vi "Create TXRX Bytes.vi"(0 "Cluster Array in":T1[](array[typedef]) {"payload" format="%x"; "timestamp" format="%<%.7X\n%x>T"; "type" items=["CAN Data"=0, "CAN Remote"=1, "CAN Bus Error"=2, "CAN 2.0 Data"=8, "CAN FD Data"=16, "CAN FD+BRS Data"=24, "J1939 Data"=192, "Delay"=224, "Log Trigger"=225, "Start Trigger"=226]; "identifier" format="%x"}, 1 "Tx?":bool) -> (7 "Array":string[](array[string]), 8 "Flow Control?":bool, 9 "Block Size":u16 format="%.0x")   [LabVIEW 2018]
uses:
  <vilib>/xnet/xnet.llb/XNET Frame CAN.ctl
  <vilib>/xnet/xnet.llb/XNET Frame Type CAN.ctl
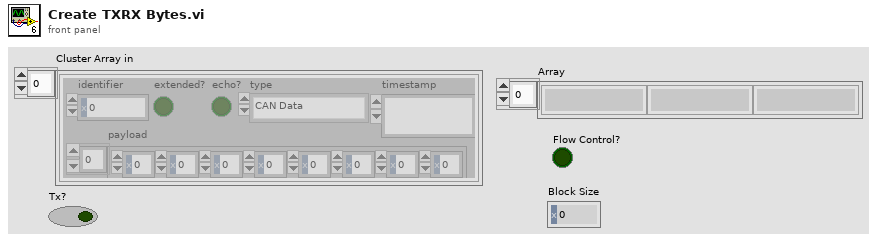
[diagram p1: front panel]
types:
  T1 = typedef "XNET Frame CAN.ctl" = cluster{"timestamp":timestamp, "payload":u8[], "identifier":u32, "type":T2, "extended?":bool, "echo?":bool}
  T2 = typedef "XNET Frame Type CAN.ctl" = u8
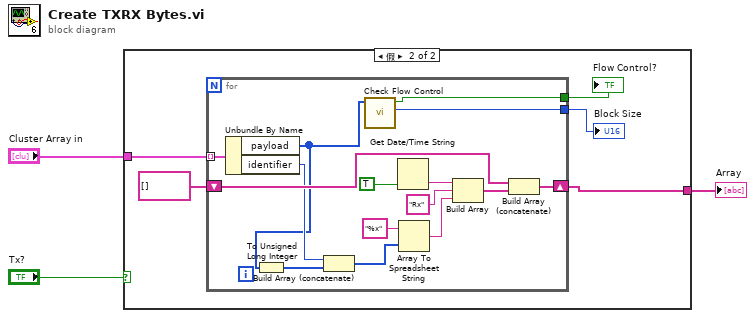
[diagram p0: block diagram]
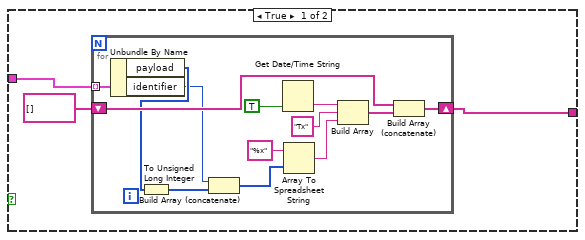
[diagram p2: hidden frame]
diagram:
  n1 = case shown="假" "Tx?" {
    tunnel: [w6 w24] -> w3
    tunnel: "Cluster Array in" -> [w5 w23]
    frame True {
      n2 = for {
        tunnel: w5 -> [w19] mode=indexing
        shift-right: [w11] -> w6
        shift-left: string[] [] -> [w9]
        n3 = Unbundle By Name(w19) -> ("payload"=w8:u8[], "identifier"=w7:u32)
        n4 = To Unsigned Long Integer(number=w8) -> (unsigned 32bit integer=w18:u32[])
        n5 = Build Array (concatenate)(w7, w18) -> (w13:u32[])
        n6 = Get Date/Time String(want seconds? (F)=TRUE) -> (time string=w15:string)  [unwired: 2 in, 1 out]
        n7 = Array To Spreadsheet String(array=w13, 3:"%x" ("format string")) -> (spreadsheet string=w17:string)  [unwired: 1 in]
        n8 = Build Array(w15, "Tx" ("format string"), w17) -> (w10:string[])
        n9 = Build Array (concatenate)(w9, w10) -> (w11:string[])
      }
    }
    frame False {
      n10 = for {
        tunnel: w23 -> [w39] mode=indexing
        shift-right: [w31] -> w24
        shift-left: string[] [] -> [w29]
        tunnel: [w26] -> w21
        tunnel: [w25] -> w20
        n11 = Unbundle By Name(w39) -> ("payload"=w27:u8[], "identifier"=w28:u32)
        n12 = To Unsigned Long Integer(number=w27) -> (unsigned 32bit integer=w38:u32[])
        n13 = Build Array (concatenate)(w28, w38) -> (w33:u32[])
        n14 = call "Check Flow Control.vi"("payload"=w27) -> ("Block Size"=w26:u16, "Flow Control?"=w25:bool)  [unwired: 9 in]
        n15 = Get Date/Time String(want seconds? (F)=TRUE) -> (time string=w35:string)  [unwired: 2 in, 1 out]
        n16 = Array To Spreadsheet String(array=w33, 3:"%x" ("format string")) -> (spreadsheet string=w37:string)  [unwired: 1 in]
        n17 = Build Array(w35, "Rx" ("format string"), w37) -> (w30:string[])
        n18 = Build Array (concatenate)(w29, w30) -> (w31:string[])
      }
      "Block Size" <- w21
      "Flow Control?" <- w20
    }
  }
  "Array" <- w3
